vi "CTRL_Send Cmd + Data.vi"(0 "Port":refnum<visa-resource-name>, 5 "RS-485 addr.":u8, 7 "Cmd":T1="D", 9 "Data":sgl, 11 "Error In":errorcluster) -> (4 "Port out":refnum<visa-resource-name>, 15 "Error Out":errorcluster)   [LabVIEW 2020]
uses:
  ctls/CTRL_Cmd.ctl
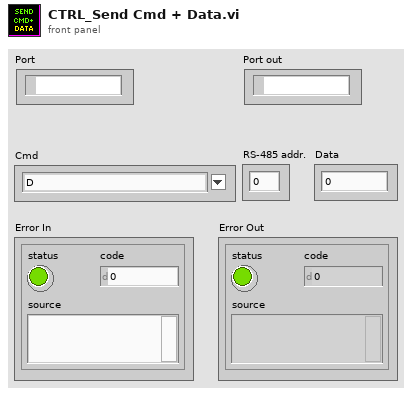
[diagram p1: front panel]
types:
  T1 = typedef "CTRL_Cmd.ctl" = string
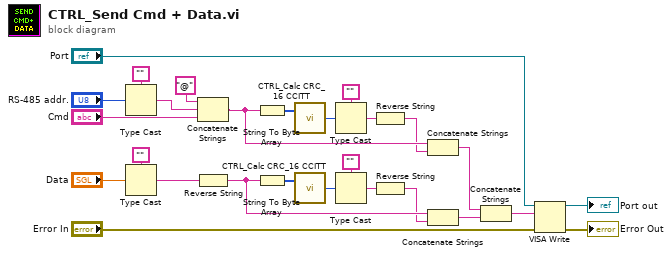
[diagram p0: block diagram]
diagram:
  n1 = Type Cast(type="", x="RS-485 addr.") -> (*(type *) &x=w16:string)
  n2 = Type Cast(type="", x="Data") -> (*(type *) &x=w20:string)
  n3 = Concatenate Strings("@", w16, "Cmd") -> (w7:string)
  n4 = Reverse String(1:w20) -> (0:w5:string)
  n5 = String To Byte Array(string=w7) -> (unsigned byte array=w10:u8[])
  n6 = String To Byte Array(string=w5) -> (unsigned byte array=w11:u8[])
  n7 = call "CTRL_Calc CRC_16 CCITT.vi"("Data bytes"=w10) -> ("CRC_16-CCITT"=w9:u16)  [unwired: 1 in]
  n8 = call "CTRL_Calc CRC_16 CCITT.vi"("Data bytes"=w11) -> ("CRC_16-CCITT"=w12:u16)  [unwired: 1 in]
  n9 = Type Cast(type="", x=w9) -> (*(type *) &x=w4:string)
  n10 = Type Cast(type="", x=w12) -> (*(type *) &x=w2:string)
  n11 = Reverse String(1:w4) -> (0:w3:string)
  n12 = Reverse String(1:w2) -> (0:w1:string)
  n13 = Concatenate Strings(w7, w3) -> (w14:string)
  n14 = Concatenate Strings(w5, w1) -> (w15:string)
  n15 = Concatenate Strings(w14, w15) -> (w6:string)
  n16 = VISA Write(VISA resource name="Port", write buffer=w6, error in (no error)="Error In") -> (VISA resource name out=→"Port out":refnum<visa-resource-name>, error out=→"Error Out":errorcluster)  [unwired: 1 out]
